vi "DAQmx_AO_LED_Switch.vi"() -> ()   [LabVIEW 2015]
panel:
  in  "Text Ring":u16(ring) items=["On"=3, "off"=0]
  in  "Stop Button":bool
  in  "device name":tag="Dev4"
  in  "stop (F)":bool
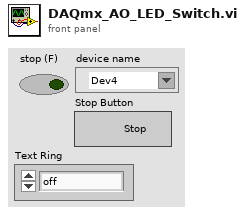
[diagram p1: front panel]
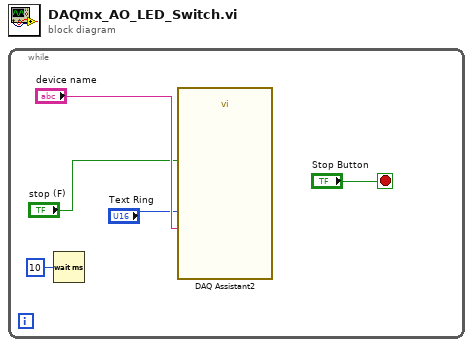
[diagram p0: block diagram]
diagram:
  n1 = while {
    stop <- "Stop Button" stop-if-true
    n2 = Wait (ms)(milliseconds to wait=u32 10) -> ()  [unwired: 1 out]
    n3 = call "DAQ Assistant2"("data"="Text Ring", "stop (T)"="stop (F)", "device name"="device name") -> ()  [unwired: 15 in, 2 out]
  }
